vi "TestAdm_ResultString.vi"(1 "Sequence start time":string, 2 "Nr of steps":i32, 3 "Nr of PASS":i32) -> (16 "Result string":string)   [LabVIEW 2020]
doc: "Create result string."
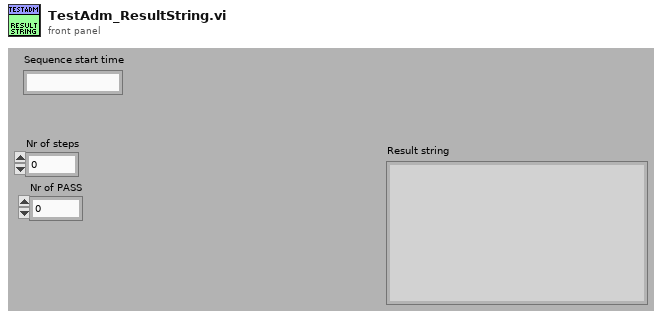
[diagram p1: front panel]
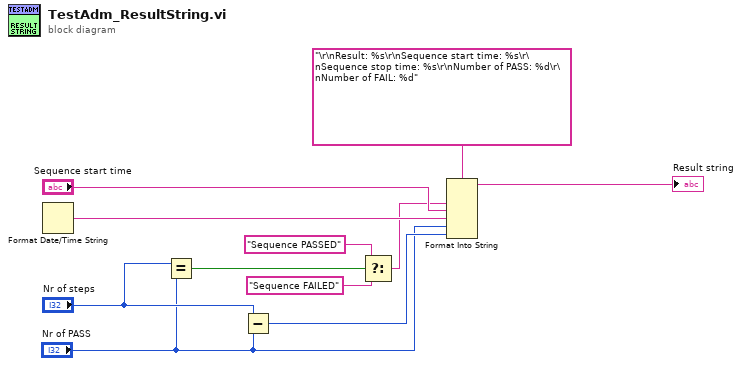
[diagram p0: block diagram]
diagram:
  n1 = Format Date/Time String() -> (date/time string=w5:string)  [unwired: 3 in]
  n2 = Equal?(x="Nr of steps", y="Nr of PASS") -> (x = y?=w3:bool)
  n3 = Subtract(x="Nr of steps", y="Nr of PASS") -> (x-y=w7:i32)
  n4 = Select(t="Sequence PASSED", s=w3, f="Sequence FAILED") -> (s? t:f=w4:string)
  n5 = Format Into String(format string="\r\nResult: %s\r\nSequence start time: %s\r\nSequence stop time: %s\r\nNumber of PASS: %d\r\nNumber of FAIL: %d" ("Format String"), w4, "Sequence start time", w5, "Nr of PASS", w7) -> (resulting string=→"Result string":string)  [unwired: 2 in, 1 out]
